vi "CALC_MARK_FORM.vi"(0 "VISA IN":refnum<visa-resource-name>, 1 "Marker number":i32, 2 "Measurement Format":string, 5 "error in":errorcluster, 7 "Channel":i32) -> (14 "VISA Out":refnum<visa-resource-name>, 19 "error out":errorcluster)   [LabVIEW 2018, in "PNA-X.lvlib"]
doc: "CALCulate<cnum>:MARKer<mkr>:FORMat <char> \n1531\n\n(Read-Write) Sets the format of the data that will be returned in a marker data query \nCALC:MARK:Y? and the displayed value of the marker readout. The selection does not have to be \nthe same as the measurement's display format. \nSee Critical Note \nParameters \n<cnum> Channel number of the measurement. There must be a selected measurement \non that channel. If unspecified, <cnum> is set to 1. \n<mkr> Any marker number from 1 to 10; if unspecified, value is set to 1 \n<char> Choose from: \nDEFault - The format of the selected measurement \nMLINear - Linear magnitude \nMLOGarithmic - Logarithmic magnitude \nIMPedance - (R+jX) \nADMittance - (G+jB) \nPHASe - Phase \nIMAGinary - Imaginary part (Im) \nREAL - Real part (Re) \nPOLar - (Re, Im) \nGDELay - Group Delay \nLINPhase - Linear Magnitude and Phase \nLOGPhase - Log Magnitude and Phase \nExamples CALC:MARK:FORMat MLIN \ncalculate2:marker8:format Character \nQuery Syntax CALCulate<cnum>:MARKer<mkr>:FORMat? \nReturn Type Character \nDefault DEFault"
uses:
  PNA-X.lvlib
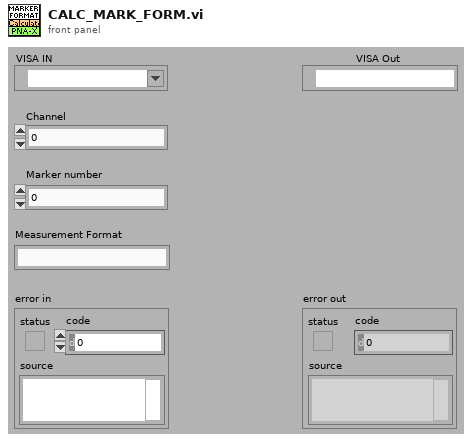
[diagram p1: front panel]
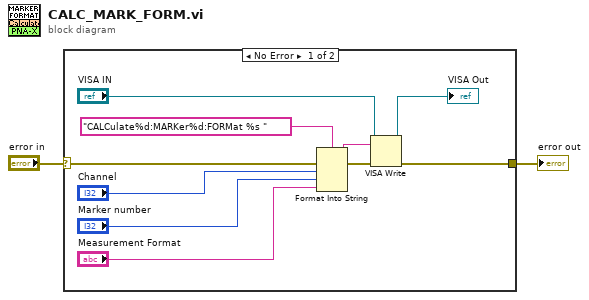
[diagram p0: block diagram]
diagram:
  n1 = case shown="No Error" "error in" {
    selector: "error in" -> [w12 w13]
    tunnel: [w7 w13] -> w1
    frame No Error {
      n2 = Format Into String(format string="CALCulate%d:MARKer%d:FORMat %s " ("Cmdline"), error in=w12, "Channel", "Marker number", "Measurement Format") -> (resulting string=w10:string, error out=w11:errorcluster)  [unwired: 1 in]
      n3 = VISA Write(VISA resource name="VISA IN", write buffer=w10, error in (no error)=w11) -> (VISA resource name out=→"VISA Out":refnum<visa-resource-name>, error out=w7:errorcluster)  [unwired: 1 out]
    }
    frame Error {
    }
  }
  "error out" <- w1
